vi "set_in_plane_move_speeds.vi"(4 "Switch X and Y (f)":bool, 6 "Echo Mode":i32, 7 "Use standard V_max (t)":bool=TRUE, 8 "error in (no error)":errorcluster, 9 "rotate by (degrees)":dbl, 10 "V_max total":dbl=15000.0, 11 "VISA resource name":refnum<visa-resource-name>) -> (0 "error out":errorcluster={"status"=FALSE, "code"=1073676294, "source"="VISA Read in write_read.vi"}, 1 "V_max Motor 2":i32, 2 "V_max Motor 1":i32, 3 "VISA ressource out":refnum<visa-resource-name>, 5 "Angle Sample Holder":dbl)   [LabVIEW 2018]
uses:
  ConversionAndInformation/Unit_Control.ctl
  MCode_LV_86/Set Parameter.ctl
panel:
  in  "Microsteps (MS=64)":dbl=64.0
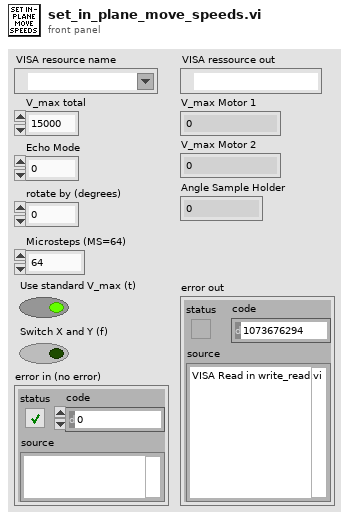
[diagram p1: front panel]
types:
  T1 = typedef "Set Parameter.ctl" = enum16{"Acceleration (A)", "Baud Rate (BD)", "Counter 1 (C1)", "Counter 2 (C2)", "Control C Software Reset (CE)", "Check Sum Enable (CK)", "Clock Mode (CM)", "Clock Mode Ratio (CR)", "Clock Mode Out Step Width (CW)", "Deceleration (D)", "Digital Filtering, Input 1 (D1)", "Digital Filtering, Input 2 (D2)", "Digital Filtering, Input 3 (D3)", "Digital Filtering, Input 4 (D4)", "Digital Filtering, Input 5 (D5)", "Digital Filtering, Input 9 (D9)", "Digital Filtering, Input 10 (D10)", "Digital Filtering, Input 11 (D11)", "Digital Filtering, Input 12 (D12)", "Deadband (DB)", "Decrement Variable (DC)", "Enable/Disable Drive (DE)", "Device Name (DN)", "End Program Execution (E)", "Encoder Function Enable (EE)", "Error Flag (EF)", "Encoder Lines (EL)", "Echo Mode (EM)", "Error Value (ER)", "Escape (ES)", "Execute Program at Address (EX)", "Firmware Version (VR)", "Hold (H)", "Hold Current (HC)", "Hold Current Delay Time (HI)", "Home to Encoder Index (HM)", "Home to Home Switch (HT)", "Increment Variable (IC)", "Initialize Parameters to NVM (IP)", "Input into Variable (IV)", "Jog Enable (JE)", "Limit Stop Mode (LM)", "Move Absolute (MA)", "Move Relative (MR)", "MicroStepping Select (MS)", "Motor Settling Delay Time (MT)", "Moving [Flag] (MV)", "Output 1 (O1)", "Output 2 (O2)", "Output 3 (O3)", "Output 4 (O4)", "Output 9 (O9)", "Output 10 (O10)", "Output 11 (O11)", "Output 12 (O12)", "Output High Byte (9-12) (OH)", "Output Low Byte (1-4) (OL)", "Output Total (1-4 and 9-12) (OT)", "Position (P)", "Position Maintenance (PM)", "Party Mode (PY)", "Register 1 (R1)", "Register 2 (R2)", "Register 3 (R3)", "Register 4 (R4)", "Reset Error(\\03)", "Run Current (RC)", "Stall Factor (SF)", "Slew (SL)", "Stall Mode Set (SM)", "Upgrade Firmware (UG)", "Velocity Initial (VI)", "Velocity Maximum (VM)", "Current1 (I1)", "Current2 (I2)", "Current3 (I3)", "Current4 (I4)", "Current5 (I5)", "Current6 (I6)", "Save (S)"}
  T2 = typedef "Unit_Control.ctl" = enum16{"Angle (Degrees)", "Rad", "Angle [TMC]", "Microsteps [TMC]", "Inches", "Nanometer", "Meter", "Centimeter", "Millimeter", "Micron"}
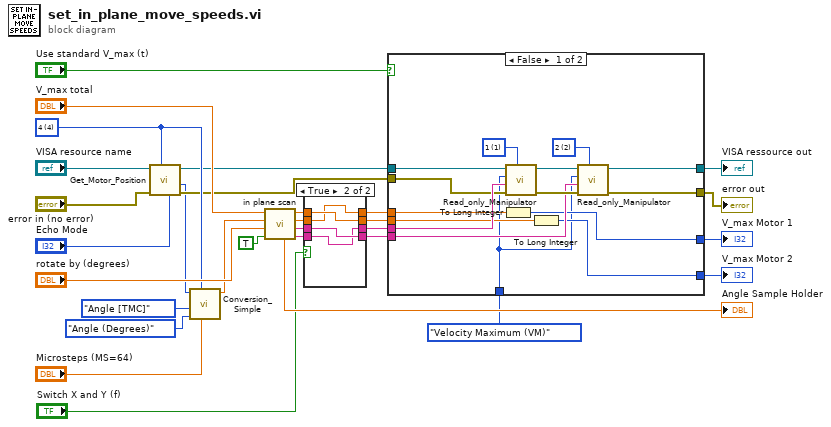
[diagram p0: block diagram]
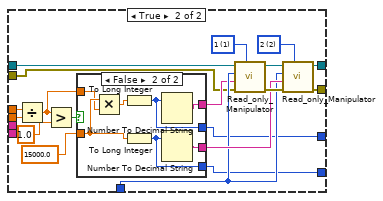
[diagram p3: hidden frame]
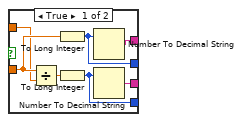
[diagram p4: hidden frame]
diagram:
  w18 = u16 4 items=["none", "1", "2", "3", "4", "all"] ("Motor")
  n1 = call "Get_Motor_Position.vi"("Echo Mode (2)"="Echo Mode", "Motor In"=w18, "error in (no error)"="error in (no error)", "VISA resource name"="VISA resource name") -> ("error out"=w16:errorcluster, "Position (Steps)"=w14:i32, "VISA ressource out"=w17:refnum<visa-resource-name>)  [unwired: 4 in, 1 out]
  n2 = call "Conversion_Simple.vi"("Microsteps (MS=64)"="Microsteps (MS=64)", "Motor"=w18, "Output Unit"=Unit_Control."Angle (Degrees)" ("Input Unit"), "Input Unit"=Unit_Control."Angle [TMC]", "Input"=w14) -> ("Output"=w20:dbl)  [unwired: 5 in, 1 out]
  n3 = call "in plane scan.vi"("abs(x,y)"=TRUE, "rotate by (degrees)"="rotate by (degrees)", "angle (degrees)"=w20, "v total"="V_max total") -> ("v_y string"=w3:string, "v_x string"=w5:string, "v_y"=w7:dbl, "v_x"=w9:dbl, "rotated angle"=→"Angle Sample Holder":dbl)  [unwired: 2 in, 1 out]
  n4 = case shown="True" "Switch X and Y (f)" {
    tunnel: w9 -> [w34 w36]
    tunnel: [w34 w35] -> w8
    tunnel: w7 -> [w33 w35]
    tunnel: [w33 w36] -> w6
    tunnel: w5 -> [w32 w38]
    tunnel: [w32 w37] -> w4
    tunnel: w3 -> [w31 w37]
    tunnel: [w31 w38] -> w2
    frame False {
    }
    frame True {
    }
  }
  n5 = case shown="False" "Use standard V_max (t)" {
    tunnel: w4 -> [w51 _]
    tunnel: w2 -> [w50 _]
    tunnel: [w47 w68] -> w28
    tunnel: [w46 w66] -> w27
    tunnel: w8 -> [w45 w65]
    tunnel: [w44 w56] -> w24
    tunnel: w6 -> [w43 w64]
    tunnel: [w42 w55] -> w23
    tunnel: w17 -> [w41 w69]
    tunnel: w16 -> [w40 w54]
    tunnel: Set_Parameter."Velocity Maximum (VM)" ("Command") -> [w39 w58]
    frame False {
      w49 = u16 1 items=["none", "1", "2", "3", "4", "all"] ("Motor")
      w48 = u16 2 items=["none", "1", "2", "3", "4", "all"] ("Motor")
      n6 = To Long Integer(number=w45) -> (32bit integer=w44:i32)
      n7 = call "Read_only_Manipulator.vi"("Motor"=w49, "error in (no error)"=w40, "Value"=w51, "Command"=w39, "VISA resource name"=w41) -> ("error out"=w53:errorcluster, "VISA ressource out"=w52:refnum<visa-resource-name>)  [unwired: 3 in, 2 out]
      n8 = To Long Integer(number=w43) -> (32bit integer=w42:i32)
      n9 = call "Read_only_Manipulator.vi"("Motor"=w48, "error in (no error)"=w53, "Value"=w50, "Command"=w39, "VISA resource name"=w52) -> ("error out"=w46:errorcluster, "VISA ressource out"=w47:refnum<visa-resource-name>)  [unwired: 3 in, 2 out]
    }
    frame True {
      w71 = u16 1 items=["none", "1", "2", "3", "4", "all"] ("Motor")
      w70 = u16 2 items=["none", "1", "2", "3", "4", "all"] ("Motor")
      n10 = Divide(x=w65, y=w64) -> (x/y=w61:dbl)
      n11 = Greater?(x=w61, y=1.0) -> (0:w62:bool)
      n12 = case shown="False" w62 {
        tunnel: w61 -> [w75 w83]
        tunnel: 15000.0 -> [w76 w84]
        tunnel: [w79 w86] -> w57
        tunnel: [w78 w85] -> w59
        tunnel: [w74 w81] -> w56
        tunnel: [w73 w80] -> w55
        frame True {
          n13 = Divide(x=w76, y=w75) -> (x/y=w77:dbl)
          n14 = To Long Integer(number=w76) -> (32bit integer=w74:i32)
          n15 = To Long Integer(number=w77) -> (32bit integer=w73:i32)
          n16 = Number To Decimal String(number=w74) -> (decimal integer string=w79:string)  [unwired: 1 in]
          n17 = Number To Decimal String(number=w73) -> (decimal integer string=w78:string)  [unwired: 1 in]
        }
        frame False {
          n18 = Multiply(x=w84, y=w83) -> (x*y=w82:dbl)
          n19 = To Long Integer(number=w82) -> (32bit integer=w81:i32)
          n20 = To Long Integer(number=w84) -> (32bit integer=w80:i32)
          n21 = Number To Decimal String(number=w81) -> (decimal integer string=w86:string)  [unwired: 1 in]
          n22 = Number To Decimal String(number=w80) -> (decimal integer string=w85:string)  [unwired: 1 in]
        }
      }
      n23 = call "Read_only_Manipulator.vi"("Motor"=w71, "error in (no error)"=w54, "Value"=w57, "Command"=w58, "VISA resource name"=w69) -> ("error out"=w67:errorcluster, "VISA ressource out"=w72:refnum<visa-resource-name>)  [unwired: 3 in, 2 out]
      n24 = call "Read_only_Manipulator.vi"("Motor"=w70, "error in (no error)"=w67, "Value"=w59, "Command"=w58, "VISA resource name"=w72) -> ("error out"=w66:errorcluster, "VISA ressource out"=w68:refnum<visa-resource-name>)  [unwired: 3 in, 2 out]
    }
  }
  "VISA ressource out" <- w28
  "error out" <- w27
  "V_max Motor 1" <- w24
  "V_max Motor 2" <- w23
